vi "MultiChannelExample.vi"() -> ()   [LabVIEW 2025]
uses:
  PalmSens/PalmSens.lvclass
  E:/PSCode/PalmSens_SDK/labview/PalmSens/Libraries/PalmSens.Core.Simplified.LabVIEW.dll
  PalmSens/Libraries/PalmSens.Core.Simplified.LabVIEW.dll
  PalmSens/MeasurementsResult.ctl
  PalmSens/MeasurementResults.ctl
  PalmSens/LiveCurveResult.ctl
panel:
  out "Measurements":T1
  out "Array 2":string[](array[string])
  out "Is Measuring 2":bool
  in  "PalmSens.lvclass 2":refnum<class "PalmSens.lvclass">
  out "LSV Method Indicator":refnum<k24>
  out "Array":string[](array[string])
  out "Is Measuring":bool
  in  "PalmSens.lvclass":refnum<class "PalmSens.lvclass">
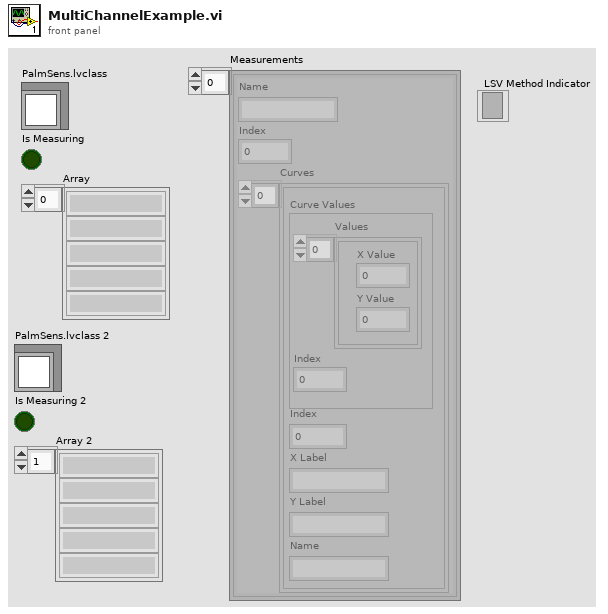
[diagram p1: front panel]
types:
  T1 = typedef "MeasurementsResult.ctl" = cluster{"Name":string, "Curves":T2, "Index":i32}[]
  T2 = typedef "MeasurementResults.ctl" = T3[]
  T3 = typedef "LiveCurveResult.ctl" = cluster{"X Label":string, "Y Label":string, "Name":string, "Index":i16, "Curve Values":cluster{"Values":cluster{"X Value":dbl, "Y Value":dbl}[], "Index":i16}}
  T4 = typedef "ActiveMeasurementInfo.ctl" = cluster{"Active Measurement":refnum<k24>, "Is Measuring Refnum":refnum<vi>, "Live Curve Result Refnum":refnum<vi>}
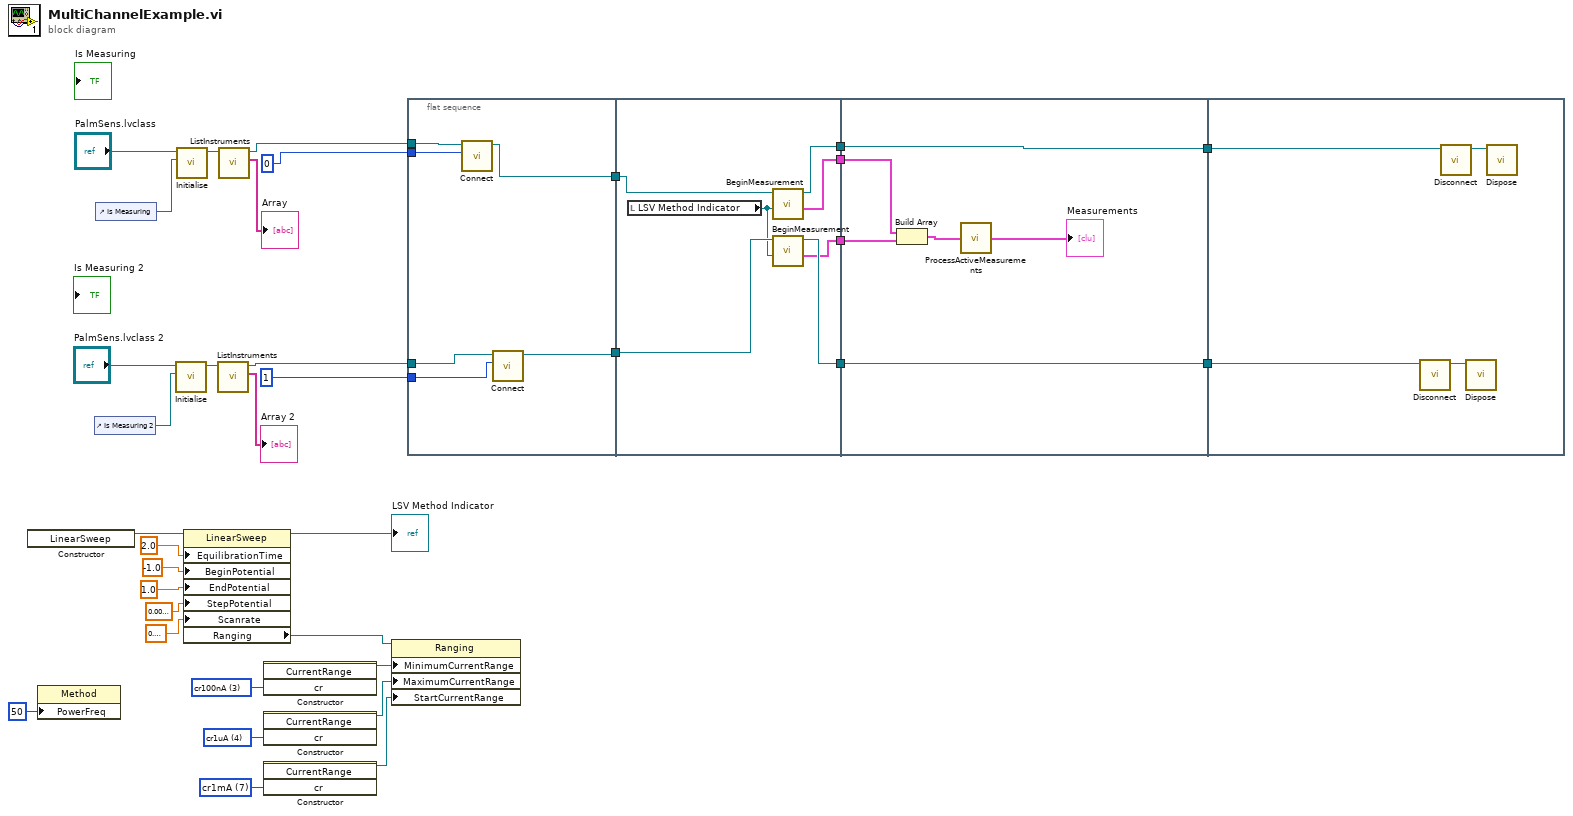
[diagram p0: block diagram]
diagram:
  w28 = 4 items=["cr100pA"=0, "cr1nA"=1, "cr10nA"=2, "cr100nA"=3, "cr1uA"=4, "cr10uA"=5, "cr100uA"=6, "cr1mA"=7, "cr10mA"=8, "cr100mA"=9, "cr2uA"=10, "cr4uA"=11, "cr8uA"=12, "cr16uA"=13, "cr32uA"=14, "cr125uA"=17, "cr250uA"=18, "cr500uA"=19, "cr5mA"=20, "cr6uA"=21, "cr13uA"=22, "cr25uA"=23, "cr50uA"=24, "cr200uA"=25, "cr63uA"=26] ("cr")
  w29 = 7 items=["cr100pA"=0, "cr1nA"=1, "cr10nA"=2, "cr100nA"=3, "cr1uA"=4, "cr10uA"=5, "cr100uA"=6, "cr1mA"=7, "cr10mA"=8, "cr100mA"=9, "cr2uA"=10, "cr4uA"=11, "cr8uA"=12, "cr16uA"=13, "cr32uA"=14, "cr125uA"=17, "cr250uA"=18, "cr500uA"=19, "cr5mA"=20, "cr6uA"=21, "cr13uA"=22, "cr25uA"=23, "cr50uA"=24, "cr200uA"=25, "cr63uA"=26] ("cr")
  w31 = 3 items=["cr100pA"=0, "cr1nA"=1, "cr10nA"=2, "cr100nA"=3, "cr1uA"=4, "cr10uA"=5, "cr100uA"=6, "cr1mA"=7, "cr10mA"=8, "cr100mA"=9, "cr2uA"=10, "cr4uA"=11, "cr8uA"=12, "cr16uA"=13, "cr32uA"=14, "cr125uA"=17, "cr250uA"=18, "cr500uA"=19, "cr5mA"=20, "cr6uA"=21, "cr13uA"=22, "cr25uA"=23, "cr50uA"=24, "cr200uA"=25, "cr63uA"=26] ("cr")
  n1 = constructor class="LinearSweep"() -> (reference out=w27:refnum<k24>)  [unwired: 3 in, 2 out]
  n2 = property class="Method"("PowerFreq"=50) -> ()  [unwired: 2 in, 2 out]
  n3 = control-ref of="Is Measuring 2"() -> (w23:refnum<vi>)
  n4 = control-ref of="Is Measuring"() -> (w34:refnum<vi>)
  n5 = call-dynamic "Initialise.vi"("Is Measuring Refnum"=w23, "PalmSens in"="PalmSens.lvclass 2") -> ("PalmSens out"=w22:refnum<class "PalmSens.lvclass">)  [unwired: 8 in, 1 out]
  n6 = call-dynamic "Initialise.vi"("Is Measuring Refnum"=w34, "PalmSens in"="PalmSens.lvclass") -> ("PalmSens out"=w33:refnum<class "PalmSens.lvclass">)  [unwired: 8 in, 1 out]
  n7 = property class="LinearSweep"(reference=w27, "EquilibrationTime"=sgl 2.0, "BeginPotential"=sgl -1.0, "EndPotential"=sgl 1.0, "StepPotential"=sgl 0.01, "Scanrate"=sgl 0.2) -> (reference out=→"LSV Method Indicator":refnum<k24>, "Ranging"=w6:refnum<k24>)  [unwired: 1 in, 1 out]
  n8 = call-dynamic "ListInstruments.vi"("PalmSens in"=w22) -> ("Array"=→"Array 2":string[], "PalmSens out"=w11:refnum<class "PalmSens.lvclass">)  [unwired: 8 in, 1 out]
  n9 = call-dynamic "ListInstruments.vi"("PalmSens in"=w33) -> ("Array"=→"Array":string[], "PalmSens out"=w13:refnum<class "PalmSens.lvclass">)  [unwired: 8 in, 1 out]
  n10 = constructor class="CurrentRange"("cr"=w31) -> (reference out=w30:refnum<k24>)  [unwired: 3 in, 3 out]
  n11 = constructor class="CurrentRange"("cr"=w28) -> (reference out=w8:refnum<k24>)  [unwired: 3 in, 3 out]
  n12 = constructor class="CurrentRange"("cr"=w29) -> (reference out=w7:refnum<k24>)  [unwired: 3 in, 3 out]
  n13 = property class="Ranging"(reference=w6, "MinimumCurrentRange"=w30, "MaximumCurrentRange"=w8, "StartCurrentRange"=w7) -> ()  [unwired: 1 in, 2 out]
  n14 = flat-sequence {
    tunnel: [w39] -> w16
    tunnel: [w36] -> w15
    tunnel: 0 ("Instrument Index") -> [w41]
    tunnel: w13 -> [w40]
    tunnel: 1 ("Instrument Index") -> [w38]
    tunnel: w11 -> [w37]
    tunnel: [w47] -> w18
    tunnel: [w44] -> w17
    tunnel: w16 -> [w48]
    tunnel: w15 -> [w45]
    tunnel: [w46] -> w10
    tunnel: [w43] -> w9
    tunnel: [w54] -> w20
    tunnel: [w53] -> w19
    tunnel: w18 -> [w54]
    tunnel: w17 -> [w53]
    tunnel: w10 -> [w52]
    tunnel: w9 -> [w51]
    tunnel: w20 -> [w56]
    tunnel: w19 -> [w55]
    frame #0 {
      n15 = call-dynamic "Connect.vi"("Instrument Index"=w41, "PalmSens in"=w40) -> ("PalmSens out"=w39:refnum<class "PalmSens.lvclass">)  [unwired: 8 in, 1 out]
      n16 = call-dynamic "Connect.vi"("Instrument Index"=w38, "PalmSens in"=w37) -> ("PalmSens out"=w36:refnum<class "PalmSens.lvclass">)  [unwired: 8 in, 1 out]
    }
    frame #1 {
      n17 = local read "LSV Method Indicator"() -> (w42:refnum<k24>)
      n18 = call-dynamic "BeginMeasurement.vi"("Method .NET Refnum"=w42, "PalmSens in"=w48) -> ("Active Measurement Info"=w46:T4, "PalmSens out"=w47:refnum<class "PalmSens.lvclass">)  [unwired: 2 in, 2 out]
      n19 = call-dynamic "BeginMeasurement.vi"("Method .NET Refnum"=w42, "PalmSens in"=w45) -> ("Active Measurement Info"=w43:T4, "PalmSens out"=w44:refnum<class "PalmSens.lvclass">)  [unwired: 2 in, 2 out]
    }
    frame #2 {
      n20 = Build Array(w52, w51) -> (w50:T4[])
      n21 = call "ProcessActiveMeasurements.vi"("Active Measurements"=w50) -> ("Measurements"=→"Measurements":T1)
    }
    frame #3 {
      n22 = call-dynamic "Disconnect.vi"("PalmSens in"=w55) -> ("PalmSens out"=w57:refnum<class "PalmSens.lvclass">)  [unwired: 9 in, 1 out]
      n23 = call-dynamic "Disconnect.vi"("PalmSens in"=w56) -> ("PalmSens out"=w58:refnum<class "PalmSens.lvclass">)  [unwired: 9 in, 1 out]
      n24 = call-dynamic "Dispose.vi"("PalmSens in"=w57) -> ()  [unwired: 9 in, 2 out]
      n25 = call-dynamic "Dispose.vi"("PalmSens in"=w58) -> ()  [unwired: 9 in, 2 out]
    }
  }
